vi "dfd_Filter Signal by MRate Coef.vi"(0 "signal in":dbl[](array[numeric]), 1 "initH?":bool, 3 "zeroPhaseH?":bool, 5 "multirate filter":T1={"mMRate_Structure"=enum."CIC", "mMRate_Mode"=0, "mMRate_Factor"=1, "mMRate_FIRParams"={"mMRate_FIR_H"=[], "mMRate_FIR_IsNyquist?"=FALSE, "mMRate_FIR_IsSymmetric?"=FALSE}, "mMRate_CICParams"={"mMRate_CIC_#Stage"=2, "mMRate_CIC_Lag"=1, "mMRate_CIC_Type"=enum."Lowpass"}, "mMRate_Order"=1, "mMRate_Version"="1.0", "mMRate_Comments"="1.0", "mMRate_RationalFactor"={"mMRate_L"=-1, "mMRate_M"=-1}, "mMRate_Fs"=1.0, "mMRate_Quantized?"=FALSE, "mMRate_QFilterGain"=1.0, "mMRate_CoefWl"=16, "mMRate_Scaling"={"mMRate_ScaleByPowerOf2?"=FALSE, "mMRate_ScaleType"=enum."Time Domain 1-Norm"}, "mMRate_InputWl"=0, "mMRate_OutputWl"=0, "mMRate_OutputMode"=enum."Nearest", "mMRate_MultMode"=enum."Truncated", "mMRate_BitPruning"=FALSE, "mMRate_GainWl"=16, "mMRate_OutputFwl"=0, "mMRate_SumIwl"=0, "mMRate_InputIwl "=16, "mMRate_SumWl"=32, "mMRate_CoefIwl"=0} {"mMRate_SumWl" min=1 max=32 step=1; "mMRate_InputIwl" min=1 max=32 step=1; "mMRate_GainWl" min=1 max=32 step=1; "mMRate_OutputWl" min=1 max=32 step=1; "mMRate_InputWl" min=1 max=32 step=1; "mMRate_CoefWl" min=1 max=32 step=1; "mMRate_Mode" items=["Default"=-1, "No Rate Change"=0, "Interpolation"=1, "Decimation"=2, "Interpolated"=3, "Rational"=4]}, 9 "skipPoint In":i32, 11 "error in (no error)":errorcluster, 12 "state in":dbl[](array[numeric]), 13 "outputPhase":i32) -> (4 "signal out":dbl[](array[numeric]), 10 "skipPoint Out":i32, 14 "state out":dbl[](array[numeric]), 15 "error out":errorcluster)   [LabVIEW 2017, in "NI_DigFilter_Process.lvlib"]
uses:
  <vilib>/addons/Digital Filter Design/NI_DigFilter_Process.lvlib
  <vilib>/addons/Digital Filter Design/_Objects.llb/DFD Multirate Filter Obj.ctl
  <vilib>/addons/Digital Filter Design/_Objects.llb/DFD Multirate Mode.ctl
  <vilib>/addons/Digital Filter Design/_Objects.llb/DFD Coef Norm Type.ctl
  <vilib>/addons/Digital Filter Design/_Objects.llb/DFD Round-off Mode.ctl
  <vilib>/addons/Digital Filter Design/_Objects.llb/DFD FXP MRate Multiply Mode.ctl
  <vilib>/addons/Digital Filter Design/NI_DigFilterLicensed.lvlib
  <resource>/LVDFD.dll
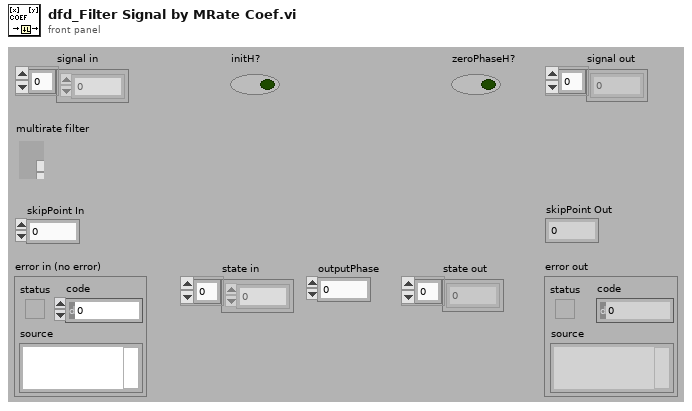
[diagram p1: front panel]
types:
  T1 = typedef "NI_DigFilterLicensed.lvlib/DFD Multirate Filter Obj.ctl" = cluster{"mMRate_Structure":enum16{"CIC", "FIR", "IIR", "Lattice"}, "mMRate_Mode":T2, "mMRate_Factor":i32, "mMRate_FIRParams":cluster{"mMRate_FIR_H":dbl[], "mMRate_FIR_IsNyquist?":bool, "mMRate_FIR_IsSymmetric?":bool}, "mMRate_CICParams":cluster{"mMRate_CIC_#Stage":i32, "mMRate_CIC_Lag":i32, "mMRate_CIC_Type":enum16{"Lowpass", "Highpass"}}, "mMRate_Order":i32, "mMRate_Version":string, "mMRate_Comments":string, "mMRate_RationalFactor":cluster{"mMRate_L":i32, "mMRate_M":i32}, "mMRate_Fs":dbl, "mMRate_Quantized?":bool, "mMRate_QFilterGain":dbl, "mMRate_CoefWl":i16, "mMRate_Scaling":cluster{"mMRate_ScaleByPowerOf2?":bool, "mMRate_ScaleType":T3}, "mMRate_InputWl":i16, "mMRate_OutputWl":i16, "mMRate_OutputMode":T4, "mMRate_MultMode":T5, "mMRate_BitPruning":bool, "mMRate_GainWl":i16, "mMRate_OutputFwl":i16, "mMRate_SumIwl":i16, "mMRate_InputIwl ":i16, "mMRate_SumWl":i16, "mMRate_CoefIwl":i16}
  T2 = typedef "NI_DigFilterLicensed.lvlib/DFD Multirate Mode.ctl" = i16
  T3 = typedef "NI_DigFilterLicensed.lvlib/DFD Coef Norm Type.ctl" = enum16{"No Norm", "Time Domain 1-Norm", "Time Domain 2-Norm", "Time Domain Inf-Norm"}
  T4 = typedef "NI_DigFilterLicensed.lvlib/DFD Round-off Mode.ctl" = enum16{"Nearest", "Truncation"}
  T5 = typedef "NI_DigFilterLicensed.lvlib/DFD FXP MRate Multiply Mode.ctl" = enum16{"Truncated", "Full"}
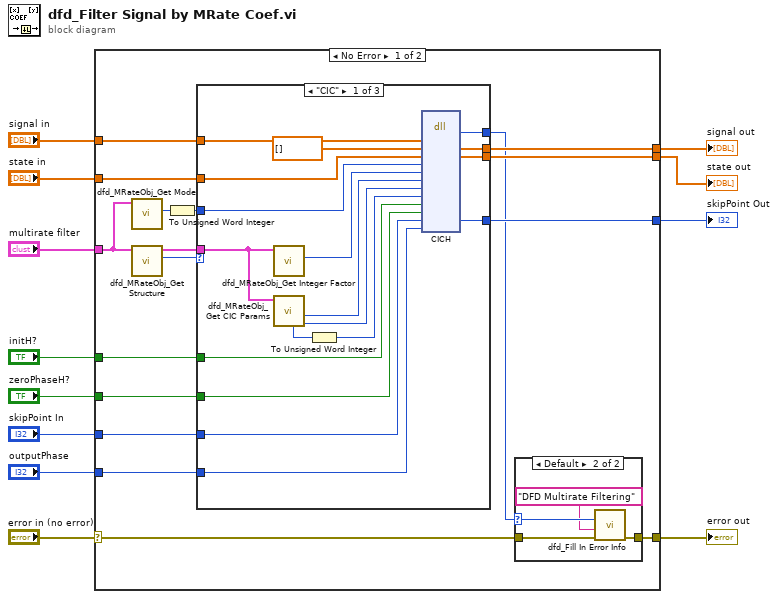
[diagram p0: block diagram]
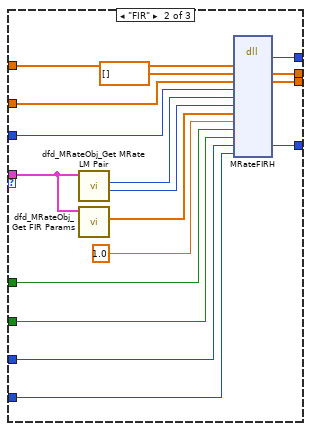
[diagram p3: hidden frame]
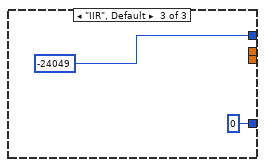
[diagram p4: hidden frame]
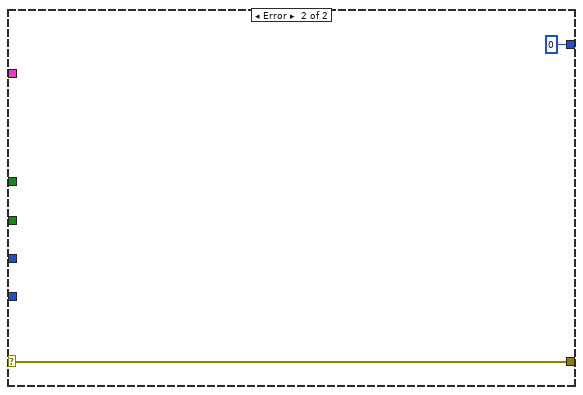
[diagram p5: hidden frame]
diagram:
  n1 = case shown="No Error" "error in (no error)" {
    selector: "error in (no error)" -> [w15 w73]
    tunnel: "multirate filter" -> [w23 _]
    tunnel: "signal in" -> [w27 _]
    tunnel: [w26 _] -> w9
    tunnel: "state in" -> [w25 _]
    tunnel: [w24 _] -> w1
    tunnel: "initH?" -> [w20 _]
    tunnel: "zeroPhaseH?" -> [w19 _]
    tunnel: "skipPoint In" -> [w18 _]
    tunnel: "outputPhase" -> [w17 _]
    tunnel: [w16 0 ("skipPoint In")] -> w3
    tunnel: [w13 w73] -> w2
    frame No Error {
      n2 = call <vilib>:"dfd_MRateObj_Get Mode.vi"("multirate filter in"=w23) -> ("mode"=w22:T2)  [unwired: 10 out]
      n3 = call <vilib>:"dfd_MRateObj_Get Structure.vi"("multirate filter in"=w23) -> ("structure"=w29:enum16{"CIC", "FIR", "IIR", "Lattice"}, "dup multirate filter"=w28:T1)  [unwired: 9 out]
      n4 = To Unsigned Word Integer(number=w22) -> (unsigned 16bit integer=w21:u16)
      n5 = case shown="\"CIC\"" w29 {
        tunnel: w28 -> [w46 w60 _]
        tunnel: w27 -> [w52 w69 _]
        tunnel: [w50 w65 _] -> w26
        tunnel: w25 -> [w49 w67 _]
        tunnel: [w48 w66 _] -> w24
        tunnel: w21 -> [w47 w64 _]
        tunnel: w20 -> [w40 w59 _]
        tunnel: w19 -> [w39 w58 _]
        tunnel: w18 -> [w38 w57 _]
        tunnel: w17 -> [w37 w56 _]
        tunnel: [w36 w55 0 ("skipPoint In")] -> w16
        tunnel: [w35 w54 -24049 ("ERR_INVALID_MULTIRATE_FILTER")] -> w14
        frame "CIC" {
          n6 = call <vilib>:"dfd_MRateObj_Get Integer Factor.vi"("multirate filter in"=w46) -> ("factor"=w45:i32)  [unwired: 10 out]
          n7 = call <vilib>:"dfd_MRateObj_Get CIC Params.vi"("multirate filter in"=w46) -> ("lag"=w43:i32, "# stages"=w44:i32, "type"=w42:enum16{"Lowpass", "Highpass"})  [unwired: 8 out]
          n8 = To Unsigned Word Integer(number=w42) -> (unsigned 16bit integer=w41:u16)
          n9 = dll-call lib="C:/Program Files/National Instruments/LabVIEW 2017/resource/LVDFD.dll" fn="CICH"("inputDataH"=w52, "outputDataH"=dbl[] [] ("signal in"), "initialStatesH"=w49, "filterModeH"=w47, "factorH"=w45, "stageH"=w44, "lagH"=w43, "filterTypeH"=w41, "initH"=w40, "zeroPhaseH"=w39, "skipPointH"=w38, "outputPhaseH"=w37) -> ("return type"=w35:i32, "outputDataH"=w50:dbl[], "initialStatesH"=w48:dbl[], "skipPointH"=w36:i32)  [unwired: 12 in, 2 out]
        }
        frame "FIR" {
          n10 = call <vilib>:"dfd_MRateObj_Get MRate LM Pair.vi"("multirate filter in"=w60) -> ("M"=w62:i32, "L"=w63:i32)  [unwired: 1 in, 8 out]
          n11 = call <vilib>:"dfd_MRateObj_Get FIR Params.vi"("multirate filter in"=w60) -> ("h(n)"=w61:dbl[])  [unwired: 10 out]
          n12 = dll-call lib="C:/Program Files/National Instruments/LabVIEW 2017/resource/LVDFD.dll" fn="MRateFIRH"("inputDataH"=w69, "outputDataH"=dbl[] [] ("signal in"), "initialStatesH"=w67, "filterModeH"=w64, "LfactorH"=w63, "MfactorH"=w62, "coefBH"=w61, "gainH"=1.0, "initH"=w59, "zeroPhaseH"=w58, "skipPointH"=w57, "outputPhaseH"=w56) -> ("return type"=w54:i32, "outputDataH"=w65:dbl[], "initialStatesH"=w66:dbl[], "skipPointH"=w55:i32)  [unwired: 12 in, 2 out]
        }
        frame "IIR", Default {
        }
      }
      n13 = case shown="Default" w14 {
        selector: w14 -> [_ w32]
        tunnel: w15 -> [w30 w34]
        tunnel: [w30 w33] -> w13
        frame 0 {
        }
        frame Default {
          n14 = call <vilib>:"dfd_Fill In Error Info.vi"("error in"=w34, "extended error info"="DFD Multirate Filtering", "status code"=w32) -> ("error out"=w33:errorcluster)  [unwired: 1 in, 7 out]
        }
      }
    }
    frame Error {
    }
  }
  "error out" <- w2
  "signal out" <- w9
  "state out" <- w1
  "skipPoint Out" <- w3
